vi "BuildSpecifications.vi"(6 "ItemBuilt":T1, 8 "error in (no error)":errorcluster, 11 "SolutionBuilder in":refnum<class "SolutionBuilder.lvclass">) -> (0 "error out":errorcluster, 3 "SolutionBuilder out":refnum<class "SolutionBuilder.lvclass">)   [LabVIEW 2020, in "SolutionBuilder.lvlib" / "SolutionBuilder.lvclass"]
uses:
  SolutionBuilder.lvclass
  BuildManager/BuildManager.lvclass
  Events/EventItemBuilt.ctl
  SolutionBuilder.lvlib
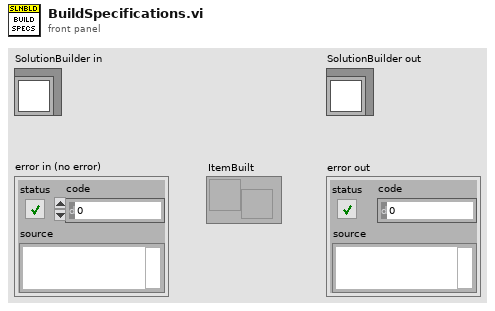
[diagram p1: front panel]
types:
  T1 = typedef "SolutionBuilder.lvlib/EventItemBuilt.ctl" = refnum<user-event>
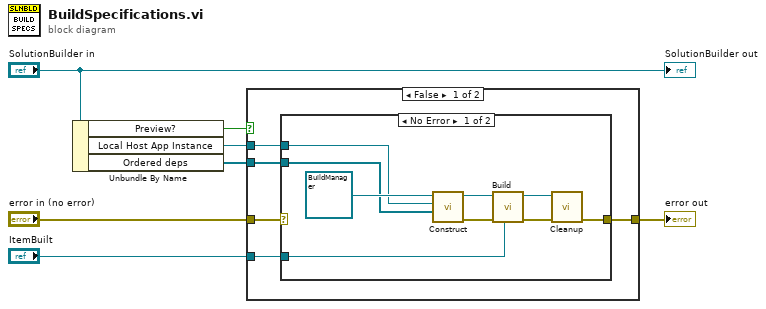
[diagram p0: block diagram]
diagram:
  n1 = Unbundle By Name("SolutionBuilder in") -> ("Preview?"=w3:bool, "Local Host App Instance"=w6:refnum<vi>, "Ordered deps"=w5:refnum<class "ProjectItem.lvclass">[])
  n2 = case shown="False" w3 {
    tunnel: w6 -> [w12 _]
    tunnel: w5 -> [w11 _]
    tunnel: "ItemBuilt" -> [w10 _]
    tunnel: "error in (no error)" -> [w9 w23]
    tunnel: [w8 w23] -> w1
    frame False {
      n3 = case shown="No Error" w9 {
        selector: w9 -> [_ w22]
        tunnel: w12 -> [w20 _]
        tunnel: w11 -> [w19 _]
        tunnel: w10 -> [w16 _]
        tunnel: [w13 w22] -> w8
        frame No Error {
          n4 = call "Construct.vi"("Ordered deps"=w19, "Application in"=w20, "BuildManager in"=refnum<class "BuildManager.lvclass"> refnum ("SolutionBuilder.lvlib:BuildManager.lvclass")) -> ("error out"=w14:errorcluster, "BuildManager out"=w18:refnum<class "BuildManager.lvclass">)  [unwired: 7 in]
          n5 = call "Build.vi"("ItemBuilt"=w16, "error in (no error)"=w14, "BuildManager in"=w18) -> ("error out"=w15:errorcluster, "BuildManager out"=w17:refnum<class "BuildManager.lvclass">)  [unwired: 7 in]
          n6 = call "Cleanup.vi"("error in (no error)"=w15, "BuildManager in"=w17) -> ("error out"=w13:errorcluster)  [unwired: 8 in, 1 out]
        }
        frame Error {
        }
      }
    }
    frame True {
    }
  }
  "error out" <- w1
  "SolutionBuilder out" <- "SolutionBuilder in"
